vi "Joystick Deadband.vi"(1 "Deadband":dbl=0.05 format="%#_13g", 2 "Joystick Value":dbl) -> (0 "Joystick Output":dbl)   [LabVIEW 2014]
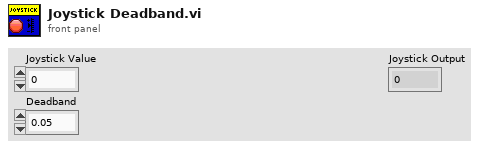
[diagram p1: front panel]
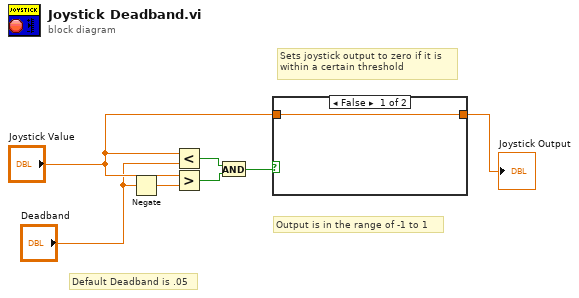
[diagram p0: block diagram]
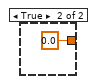
[diagram p2: hidden frame]
diagram:
  # "Output is in the range of -1 to 1"
  # "Default Deadband is .05"
  # "Sets joystick output to zero if it is \nwithin a certain threshold"
  n1 = Negate(x="Deadband") -> (-x=w2:dbl)
  n2 = Less?(x="Joystick Value", y="Deadband") -> (x < y?=w5:bool)
  n3 = Greater?(x="Joystick Value", y=w2) -> (0:w6:bool)
  n4 = And(x=w5, y=w6) -> (x .and. y?=w7:bool)
  n5 = case shown="False" w7 {
    tunnel: "Joystick Value" -> [w8 _]
    tunnel: [w8 0.0 ("Joystick Value")] -> w3
    frame False {
    }
    frame True {
    }
  }
  "Joystick Output" <- w3
